vi "Write Disconnection List.vi"(8 "error in (no error)":errorcluster, 10 "Disconnection List":string, 11 "Switch Disconnect Message in":refnum<class "Switch Disconnect Message.lvclass">) -> (0 "error out":errorcluster, 3 "Switch Disconnect Message out":refnum<class "Switch Disconnect Message.lvclass">)   [LabVIEW 2027, in "Messaging.lvlib" / "Switch Disconnect Message.lvclass"]
uses:
  Switch Disconnect Message.lvclass
  Switch Disconnect Message.lvclass/Switch Disconnect Message.ctl
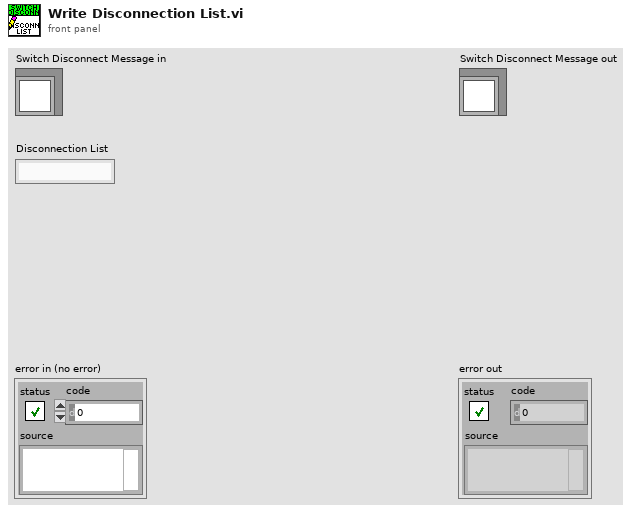
[diagram p1: front panel]
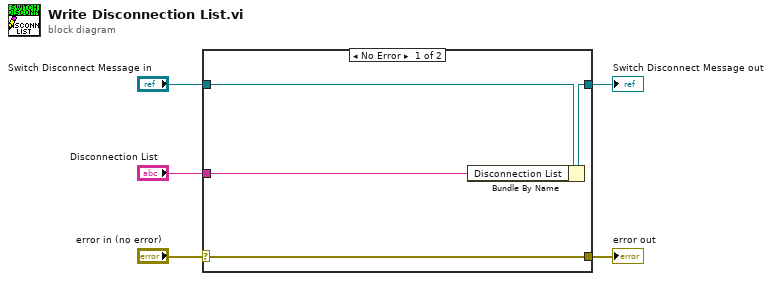
[diagram p0: block diagram]
diagram:
  n1 = case shown="No Error" "error in (no error)" {
    selector: "error in (no error)" -> [w9 w10]
    tunnel: [w9 w10] -> w4
    tunnel: [w7 w11] -> w2
    tunnel: "Switch Disconnect Message in" -> [w8 w11]
    tunnel: "Disconnection List" -> [w6 _]
    frame No Error {
      n2 = Bundle By Name(cluster=w8, "Disconnection List"=w6) -> (w7:refnum<class "Switch Disconnect Message.lvclass">)
    }
    frame Error {
    }
  }
  "error out" <- w4
  "Switch Disconnect Message out" <- w2
